vi "freqCurveTemp.vi"(0 "error in (no error)":errorcluster, 4 "Step":dbl, 5 "Path":path, 6 "End":dbl, 7 "Start":dbl) -> (1 "error out":errorcluster)   [LabVIEW 2010]
panel:
  out "WC Amplitude":dbl(graph)
  out "WC Phase Shift":dbl(graph)
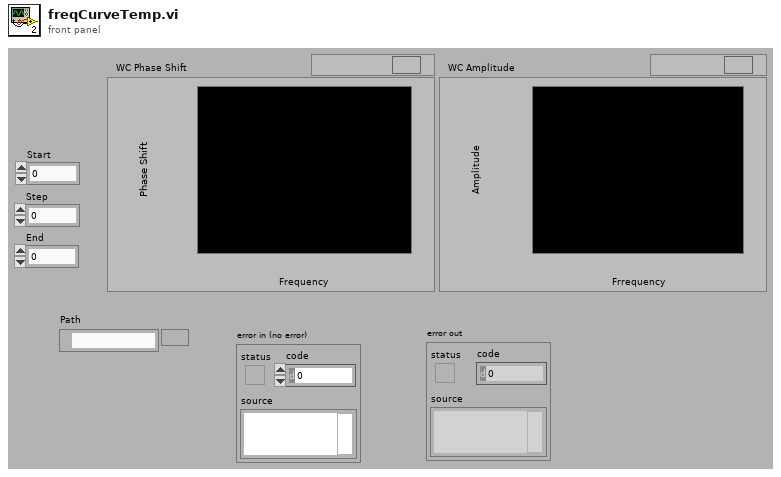
[diagram p1: front panel]
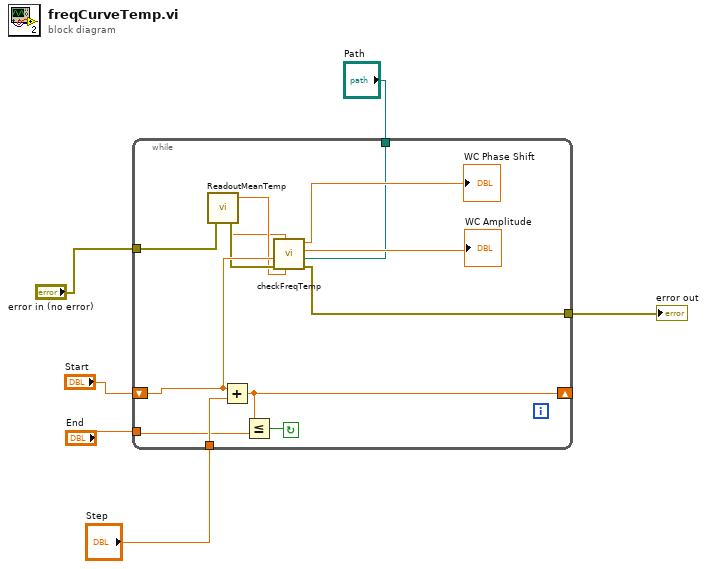
[diagram p0: block diagram]
diagram:
  n1 = while {
    shift-right: [w17] -> _
    shift-left: "Start" -> [w11]
    tunnel: "Step" -> [w19]
    tunnel: "End" -> [w16]
    tunnel: "error in (no error)" -> [w10]
    tunnel: [w12] -> w2
    tunnel: "Path" -> [w13]
    stop <- w18 continue-if-true
    n2 = call "ReadoutMeanTemp.vi"("error in (no error)"=w10) -> ("error out"=w9:errorcluster, "Error Temp"=w7:dbl, "Temperature"=w8:dbl)  [unwired: 2 in]
    n3 = Add(x=w11, y=w19) -> (x+y=w17:dbl)
    n4 = Less Or Equal?(x=w17, y=w16) -> (x <= y?=w18:bool)
    n5 = call "checkFreqTemp.vi"("Path"=w13, "Temp"=w8, "Error Temp"=w7, "error in"=w9, "Set Frequency"=w11) -> ("error out"=w12:errorcluster, "Amplitude"=→"WC Amplitude":dbl, "Phase Shift"=→"WC Phase Shift":dbl)  [unwired: 2 in]
  }
  "error out" <- w2
